vi "initialize slider tabs.vi"   [LabVIEW 2012]
uses:
  GFG/GFGbooleanGet.vi
  GFG/GFG library.lvlib
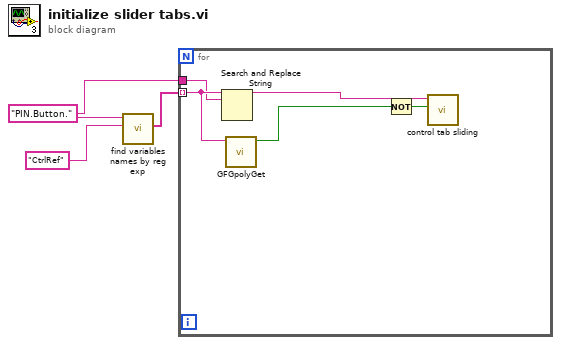
[diagram p0: block diagram]
diagram:
  w1 = "PIN.Button." ("exclude string (reg exp)")
  n1 = call "find variables  names by reg exp.vi"("exclude string (reg exp)"="CtrlRef", "search string (reg exp)"=w1) -> ("Array of Variable Names"=w3:string[])  [unwired: 8 in, 1 out]
  n2 = for {
    tunnel: w3 -> [w8] mode=indexing
    tunnel: w1 -> [w7]
    n3 = Search and Replace String(input string=w8, search string=w7) -> (result string=w6:string)  [unwired: 6 in, 3 out]
    n4 = call-poly "GFGpolyGet.vi"("Variable Name in"=w8) -> ("Boolean"=w5:bool)  [unwired: 10 in]
    n5 = Not(x=w5) -> (.not. x?=w4:bool)
    n6 = call "control tab sliding.vi"("close(T)/open(F)"=w4, "String"=w6) -> ()  [unwired: 10 in]
  }
